vi "File manager - List.vi"() -> ()   [LabVIEW 2011]
doc: "This is a <B>file manager application</B> that allows you to <B>transfer files between your computer and your Amazon S3 buckets.</B>\n\nYou can donwload, upload and delete files by selecting actions from right-click menus or using drag and drop between the panes listing local and cloud files."
uses:
  __File manager Data type.ctl
panel:
  in  "Stop":bool
  in  "Local Drives":string(combo)
  in  "Buckets":string(combo)
  in  "Cloud List":i32(listbox)
  in  "Local List":i32(listbox)
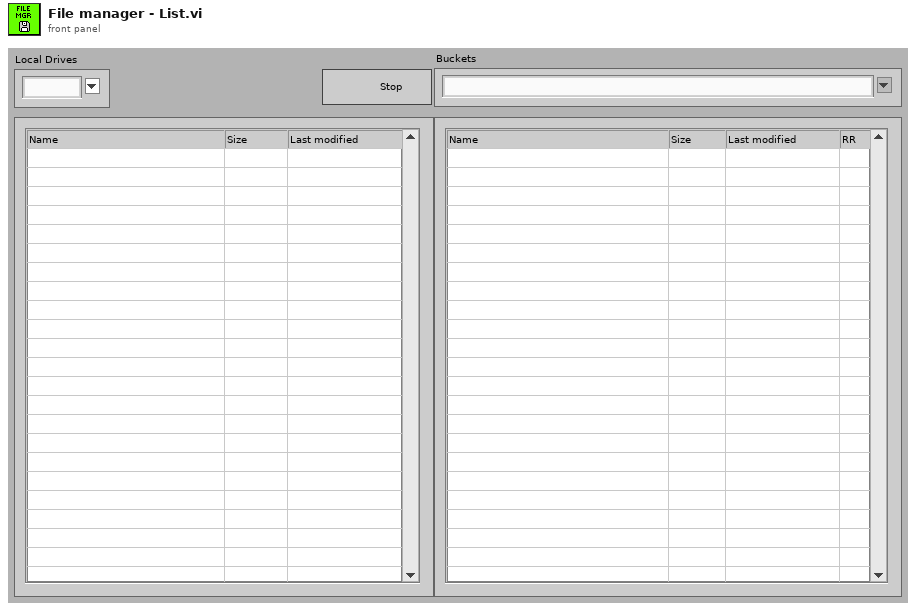
[diagram p1: front panel]
types:
  T1 = typedef "__File manager Data type.ctl" = cluster{"Drive List":refnum<vi>, "Bucket List":refnum<vi>, "Local List":refnum<vi>, "Cloud List":refnum<vi>, "Local path":path, "Cloud path":string}
  T2 = cluster{"data name":string, "drag data":variant}[]
  T3 = typedef "LVPoint32TypeDef.ctl" = cluster{"Horizontal":i32, "Vertical":i32}
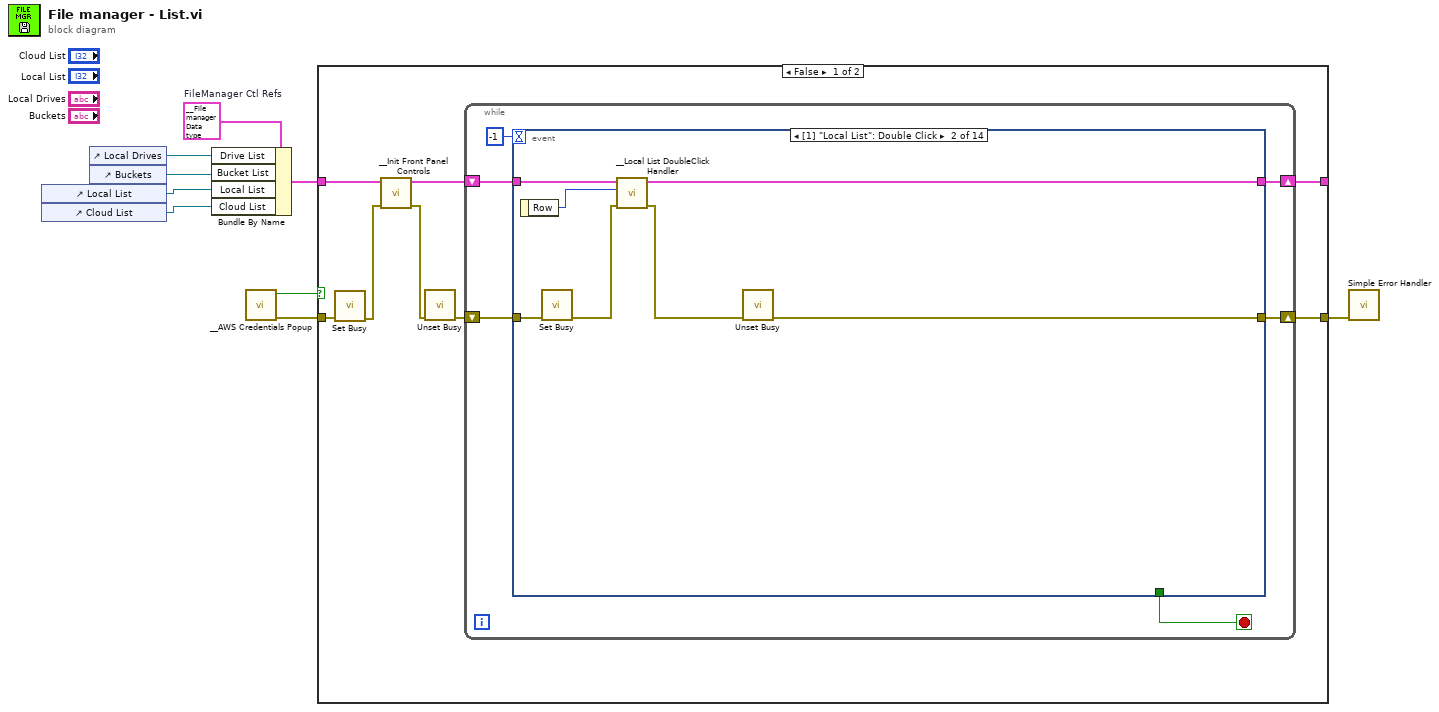
[diagram p0: block diagram]
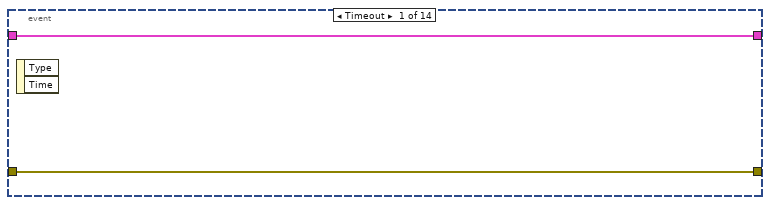
[diagram p2: hidden frame]
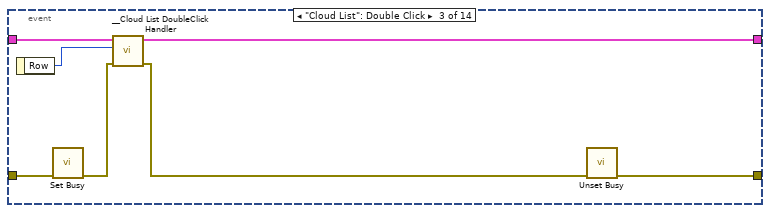
[diagram p3: hidden frame]
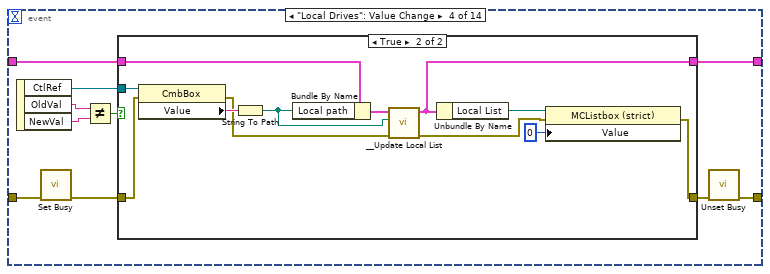
[diagram p4: hidden frame]
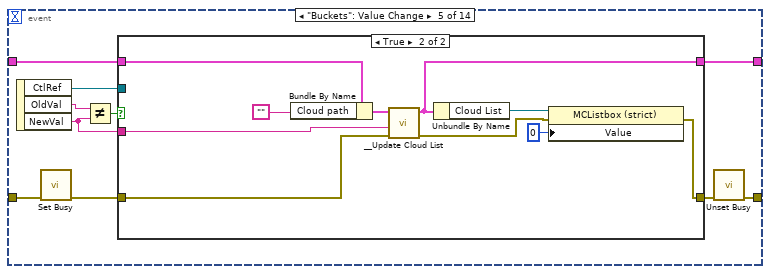
[diagram p6: hidden frame]
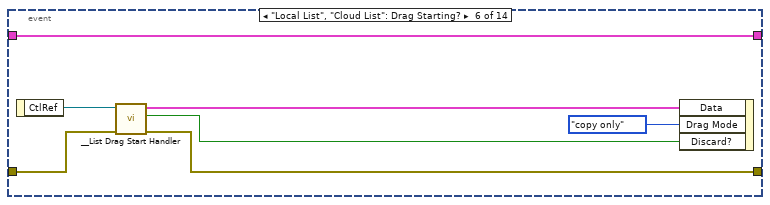
[diagram p8: hidden frame]
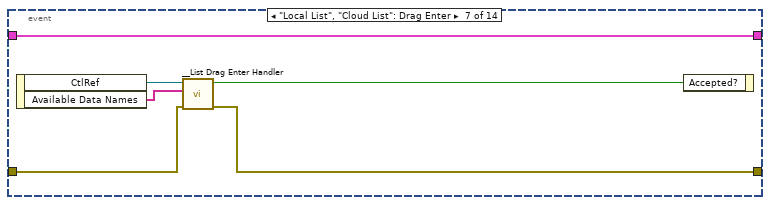
[diagram p9: hidden frame]
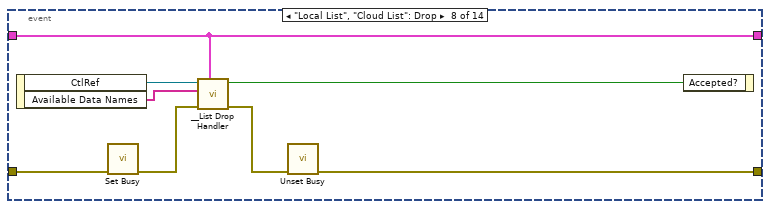
[diagram p10: hidden frame]
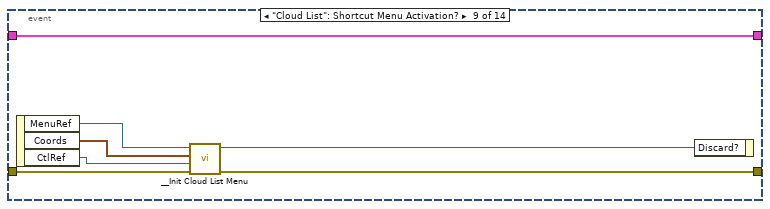
[diagram p11: hidden frame]
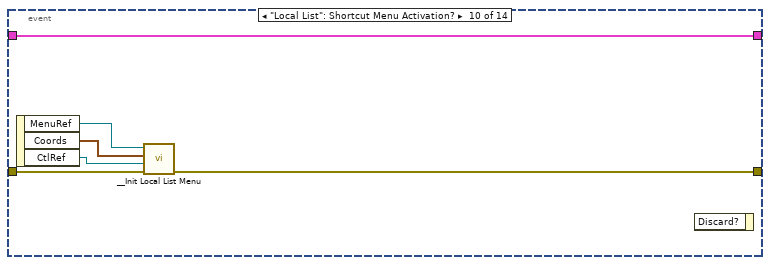
[diagram p12: hidden frame]
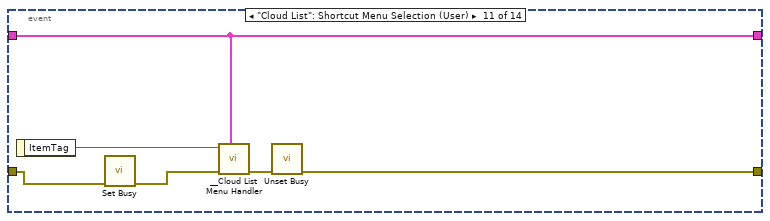
[diagram p13: hidden frame]
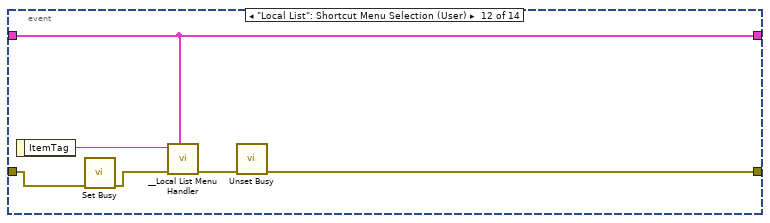
[diagram p14: hidden frame]
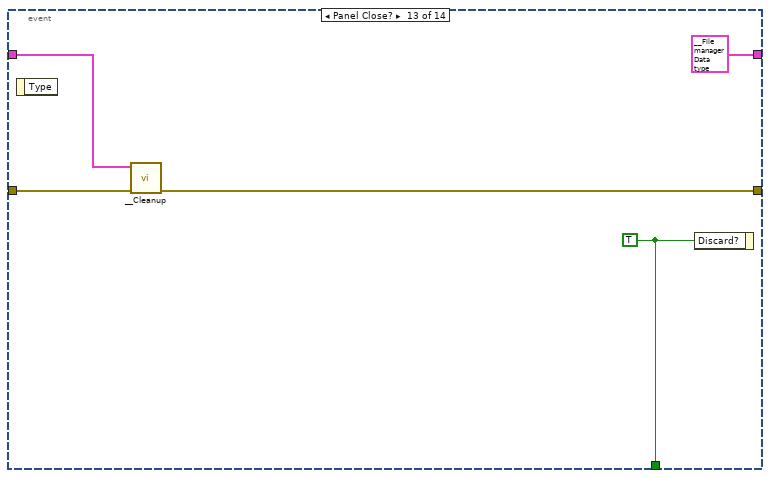
[diagram p15: hidden frame]
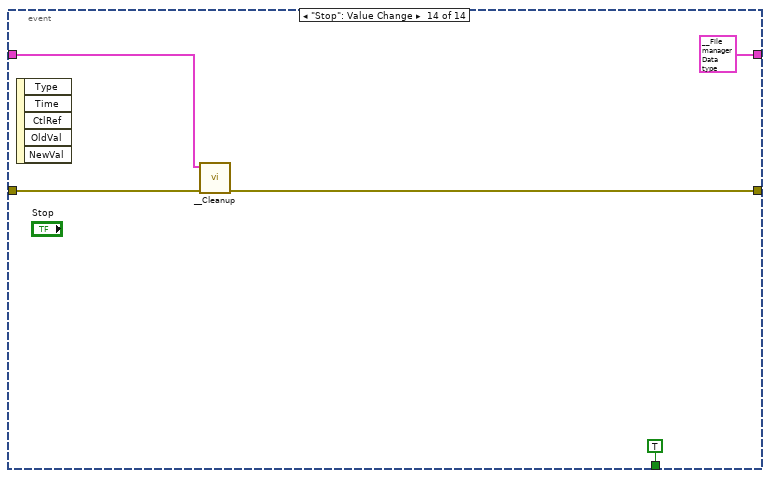
[diagram p16: hidden frame]
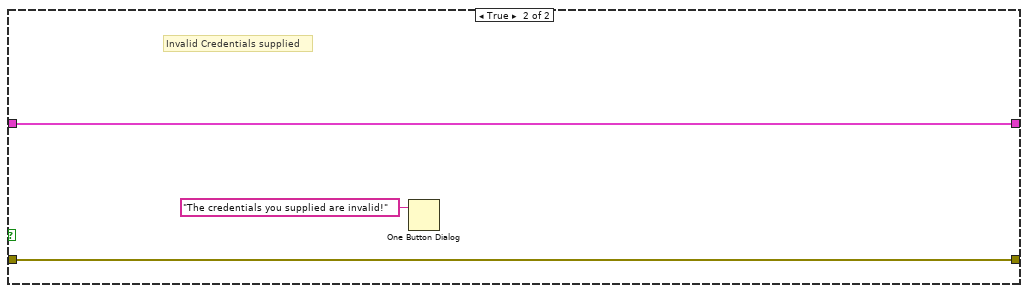
[diagram p17: hidden frame]
diagram:
  w9 = T1 {"Drive List"=refnum, "Bucket List"=refnum, "Local List"=refnum, "Cloud List"=refnum, "Local path"=path "", "Cloud path"=""}  # FileManager Ctl Refs
  n1 = control-ref of="Local List"() -> (w7:refnum<vi>)
  n2 = control-ref of="Cloud List"() -> (w6:refnum<vi>)
  n3 = control-ref of="Local Drives"() -> (w3:refnum<vi>)
  n4 = control-ref of="Buckets"() -> (w8:refnum<vi>)
  n5 = Bundle By Name(cluster=w9, "Drive List"=w3, "Bucket List"=w8, "Local List"=w7, "Cloud List"=w6) -> (w5:T1)
  n6 = call "__AWS Credentials Popup.vi"() -> ("error out"=w2:errorcluster, "Invalid Credentials"=w1:bool)  [unwired: 9 in, 1 out]
  n7 = case shown="False" w1 {
    tunnel: [w17 w143] -> w4
    tunnel: w5 -> [w15 w142]
    tunnel: w2 -> [w13 w143]
    tunnel: [w14 w142] -> _
    frame False {
      n8 = call <vilib>:"Set Busy.vi"("error in (no error)"=w13) -> ("error out"=w12:errorcluster)  [unwired: 9 in, 1 out]
      n9 = call "__Init Front Panel Controls.vi"("error in (no error)"=w12, "FileManager Ctl Refs in"=w15) -> ("error out"=w10:errorcluster, "FileManager Ctl Refs out"=w16:T1)  [unwired: 8 in]
      n10 = call <vilib>:"Unset Busy.vi"("error in (no error)"=w10) -> ("error out"=w11:errorcluster)  [unwired: 10 in]
      n11 = while {
        shift-right: [w19] -> w17
        shift-left: w11 -> [w21]
        shift-right: [w18] -> w14
        shift-left: w16 -> [w23]
        stop <- w22 stop-if-true
        n12 = event shown="[1] \"Local List\": Double Click" {
          selector: _ -> [_ _ _ _ _ _ _ _ _ _ _ _ _ _]
          dyn-events: _ -> [_ _ _ _ _ _ _ _ _ _ _ _ _ _]
          timeout: -1 -> [_ _ _ _ _ _ _ _ _ _ _ _ _ _]
          tunnel: w23 -> [w24 w32 w39 w48 w72 w87 w98 w103 w110 w114 w124 w130 w133 w138]
          tunnel: [_ _ _ _ _ _ _ _ _ _ _ _ w136 TRUE ("Discard?")] -> w22
          tunnel: w21 -> [w25 w29 w36 w43 w67 w91 w95 w102 w113 w119 w123 w129 w134 w139]
          tunnel: [w25 w26 w33 w40 w64 w90 w94 w99 w111 w115 w120 w126 w132 w137] -> w19
          tunnel: [w24 w31 w38 w47 w71 w87 w98 w103 w110 w114 w124 w130 T1 {"Drive List"=refnum, "Bucket List"=refnum, "Local List"=refnum, "Cloud List"=refnum, "Local path"=path "", "Cloud path"=""} ("FileManager Ctl Refs out") T1 {"Drive List"=refnum, "Bucket List"=refnum, "Local List"=refnum, "Cloud List"=refnum, "Local path"=path "", "Cloud path"=""} ("FileManager Ctl Refs out")] -> w18
          event Timeout {
            n13 = event-data() -> ()  [unwired: 1 in, 2 out]
          }
          event "Local List": Double Click {
            n14 = event-data() -> ("Row"=w30:i32)  [unwired: 1 in]
            n15 = call <vilib>:"Set Busy.vi"("error in (no error)"=w29) -> ("error out"=w28:errorcluster)  [unwired: 9 in, 1 out]
            n16 = call "__Local List DoubleClick Handler.vi"("error in (no error)"=w28, "Clicked Row"=w30, "FileManager Data in"=w32) -> ("error out"=w27:errorcluster, "FileManager Data out"=w31:T1)  [unwired: 7 in]
            n17 = call <vilib>:"Unset Busy.vi"("error in (no error)"=w27) -> ("error out"=w26:errorcluster)  [unwired: 10 in]
          }
          event "Cloud List": Double Click {
            n18 = event-data() -> ("Row"=w37:i32)  [unwired: 1 in]
            n19 = call <vilib>:"Set Busy.vi"("error in (no error)"=w36) -> ("error out"=w35:errorcluster)  [unwired: 9 in, 1 out]
            n20 = call "__Cloud List DoubleClick Handler.vi"("error in (no error)"=w35, "Clicked Row"=w37, "FileManager Data in"=w39) -> ("error out"=w34:errorcluster, "FileManager Data out"=w38:T1)  [unwired: 7 in]
            n21 = call <vilib>:"Unset Busy.vi"("error in (no error)"=w34) -> ("error out"=w33:errorcluster)  [unwired: 10 in]
          }
          event "Local Drives": Value Change {
            n22 = event-data() -> ("CtlRef"=w49:refnum<vi>, "OldVal"=w46:string, "NewVal"=w45:string)  [unwired: 1 in]
            n23 = call <vilib>:"Set Busy.vi"("error in (no error)"=w43) -> ("error out"=w42:errorcluster)  [unwired: 9 in, 1 out]
            n24 = Not Equal?(x=w46, y=w45) -> (x != y?=w44:bool)
            n25 = case shown="True" w44 {
              tunnel: w49 -> [_ w63]
              tunnel: w42 -> [w50 w62]
              tunnel: w48 -> [w51 w60]
              tunnel: [w51 w56] -> w47
              tunnel: [w50 w52] -> w41
              frame False {
              }
              frame True {
                n26 = property class="CmbBox"(reference=w63, error in=w62) -> (error out=w57:errorcluster, "Value"=w61:string)  [unwired: 1 out]
                n27 = String To Path(string=w61) -> (path=w58:path)
                n28 = Bundle By Name(cluster=w60, "Local path"=w58) -> (w59:T1)
                n29 = call "__Update Local List.vi"("error in (no error)"=w57, "Path to list"=w58, "FileManager Ctl Refs in"=w59) -> ("error out"=w53:errorcluster, "FileManager Ctl Refs out"=w56:T1)  [unwired: 7 in]
                n30 = Unbundle By Name(w56) -> ("Local List"=w55:refnum<vi>)
                n31 = property class="MCListbox (strict)"(reference=w55, error in=w53, "Value"=0) -> (error out=w52:errorcluster)  [unwired: 1 out]
              }
            }
            n32 = call <vilib>:"Unset Busy.vi"("error in (no error)"=w41) -> ("error out"=w40:errorcluster)  [unwired: 10 in]
          }
          event "Buckets": Value Change {
            n33 = event-data() -> ("CtlRef"=w73:refnum<vi>, "OldVal"=w70:string, "NewVal"=w68:string)  [unwired: 1 in]
            n34 = call <vilib>:"Set Busy.vi"("error in (no error)"=w67) -> ("error out"=w66:errorcluster)  [unwired: 9 in, 1 out]
            n35 = Not Equal?(x=w70, y=w68) -> (x != y?=w69:bool)
            n36 = case shown="True" w69 {
              tunnel: w73 -> [_ _]
              tunnel: w66 -> [w74 w78]
              tunnel: w72 -> [w75 w85]
              tunnel: [w75 w83] -> w71
              tunnel: [w74 w79] -> w65
              tunnel: w68 -> [_ w76]
              frame False {
              }
              frame True {
                n37 = Bundle By Name(cluster=w85, "Cloud path"="") -> (w84:T1)
                n38 = call "__Update Cloud List.vi"("error in (no error)"=w78, "Bucket"=w76, "FileManager Ctl Refs in"=w84) -> ("error out"=w80:errorcluster, "FileManager Ctl Refs out"=w83:T1)  [unwired: 7 in]
                n39 = Unbundle By Name(w83) -> ("Cloud List"=w82:refnum<vi>)
                n40 = property class="MCListbox (strict)"(reference=w82, error in=w80, "Value"=0) -> (error out=w79:errorcluster)  [unwired: 1 out]
              }
            }
            n41 = call <vilib>:"Unset Busy.vi"("error in (no error)"=w65) -> ("error out"=w64:errorcluster)  [unwired: 10 in]
          }
          event "Local List", "Cloud List": Drag Starting? {
            n42 = event-data() -> ("CtlRef"=w89:refnum<vi>)  [unwired: 1 in]
            n43 = call "__List Drag Start Handler.vi"("error in (no error)"=w91, "MCListbox Refnum"=w89) -> ("error out"=w90:errorcluster, "Discard Drag?"=w86:bool, "Drag Data"=w88:T2)  [unwired: 7 in]
            n44 = event-data("Data"=w88, "Drag Mode"=enum32{"copy or move", "copy only", "move only"}."copy only", "Discard?"=w86) -> ()  [unwired: 1 in, 1 out]
          }
          event "Local List", "Cloud List": Drag Enter {
            n45 = event-data() -> ("CtlRef"=w96:refnum<vi>, "Available Data Names"=w97:string[])  [unwired: 1 in]
            n46 = call "__List Drag Enter Handler.vi"("error in (no error)"=w95, "Available data names"=w97, "MCListbox Refnum"=w96) -> ("error out"=w94:errorcluster, "Accept?"=w93:bool)  [unwired: 7 in]
            n47 = event-data("Accepted?"=w93) -> ()  [unwired: 1 in, 1 out]
          }
          event "Local List", "Cloud List": Drop {
            n48 = event-data() -> ("CtlRef"=w106:refnum<vi>, "Available Data Names"=w105:string[])  [unwired: 1 in]
            n49 = call <vilib>:"Set Busy.vi"("error in (no error)"=w102) -> ("error out"=w101:errorcluster)  [unwired: 9 in, 1 out]
            n50 = call "__List Drop Handler.vi"("FileManager Data"=w103, "error in (no error)"=w101, "Available data names"=w105, "MCListbox Refnum"=w106) -> ("error out"=w100:errorcluster, "Accept?"=w104:bool)  [unwired: 6 in]
            n51 = call <vilib>:"Unset Busy.vi"("error in (no error)"=w100) -> ("error out"=w99:errorcluster)  [unwired: 10 in]
            n52 = event-data("Accepted?"=w104) -> ()  [unwired: 1 in, 1 out]
          }
          event "Cloud List": Shortcut Menu Activation? {
            n53 = event-data() -> ("MenuRef"=w112:refnum<k9>, "Coords"=w108:T3, "CtlRef"=w109:refnum<vi>)  [unwired: 1 in]
            n54 = call "__Init Cloud List Menu.vi"("error in (no error)"=w113, "MCListbox Refnum"=w109, "Coords"=w108, "menu reference"=w112) -> ("error out"=w111:errorcluster, "Discard?"=w107:bool)  [unwired: 6 in]
            n55 = event-data("Discard?"=w107) -> ()  [unwired: 1 in, 1 out]
          }
          event "Local List": Shortcut Menu Activation? {
            n56 = event-data() -> ("MenuRef"=w116:refnum<k9>, "Coords"=w117:T3, "CtlRef"=w118:refnum<vi>)  [unwired: 1 in]
            n57 = call "__Init Local List Menu.vi"("error in (no error)"=w119, "MCListbox Refnum"=w118, "Coords"=w117, "menu reference"=w116) -> ("error out"=w115:errorcluster)  [unwired: 6 in, 1 out]
            n58 = event-data() -> ()  [unwired: 2 in, 1 out]
          }
          event "Cloud List": Shortcut Menu Selection (User) {
            n59 = event-data() -> ("ItemTag"=w125:string)  [unwired: 1 in]
            n60 = call <vilib>:"Set Busy.vi"("error in (no error)"=w123) -> ("error out"=w122:errorcluster)  [unwired: 9 in, 1 out]
            n61 = call "__Cloud List Menu Handler.vi"("FileManager Data"=w124, "error in (no error)"=w122, "Menuitem Tag"=w125) -> ("error out"=w121:errorcluster)  [unwired: 8 in]
            n62 = call <vilib>:"Unset Busy.vi"("error in (no error)"=w121) -> ("error out"=w120:errorcluster)  [unwired: 10 in]
          }
          event "Local List": Shortcut Menu Selection (User) {
            n63 = event-data() -> ("ItemTag"=w131:string)  [unwired: 1 in]
            n64 = call <vilib>:"Set Busy.vi"("error in (no error)"=w129) -> ("error out"=w128:errorcluster)  [unwired: 9 in, 1 out]
            n65 = call "__Local List Menu Handler.vi"("FileManager Data"=w130, "error in (no error)"=w128, "Menuitem Tag"=w131) -> ("error out"=w127:errorcluster)  [unwired: 8 in]
            n66 = call <vilib>:"Unset Busy.vi"("error in (no error)"=w127) -> ("error out"=w126:errorcluster)  [unwired: 10 in]
          }
          event Panel Close? {
            w136 = TRUE ("Discard?")
            n67 = event-data() -> ()  [unwired: 1 in, 1 out]
            n68 = call "__Cleanup.vi"("error in (no error)"=w134, "FileManager Data in"=w133) -> ("error out"=w132:errorcluster)  [unwired: 9 in]
            n69 = event-data("Discard?"=w136) -> ()  [unwired: 1 in, 1 out]
          }
          event "Stop": Value Change {
            n70 = event-data() -> ()  [unwired: 1 in, 5 out]
            n71 = call "__Cleanup.vi"("error in (no error)"=w139, "FileManager Data in"=w138) -> ("error out"=w137:errorcluster)  [unwired: 9 in]
          }
        }
      }
    }
    frame True {
      # "Invalid Credentials supplied"
      n72 = One Button Dialog(message="The credentials you supplied are invalid!") -> ()  [unwired: 1 in, 1 out]
    }
  }
  n73 = call <vilib>:"Simple Error Handler.vi"("error in (no error)"=w4) -> ()  [unwired: 4 in, 5 out]
